vi "Coordinate Space Transaction Lists.vi"(4 "Coordinate Space":bool caption="Coord", 5 "error in (no error)":errorcluster, 6 "Include Command":bool, 7 "Source":T1, 8 "Include Reading":bool) -> (0 "error out":errorcluster, 3 "Transactions":string[](array[string]))   [LabVIEW 2013]
uses:
  Names/Source Group Type.ctl
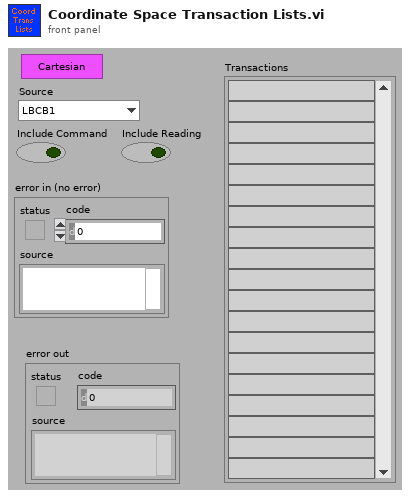
[diagram p1: front panel]
types:
  T1 = typedef "Source Group Type.ctl" = enum16{"LBCB1", "LBCB2", "Consolidated", "External"}
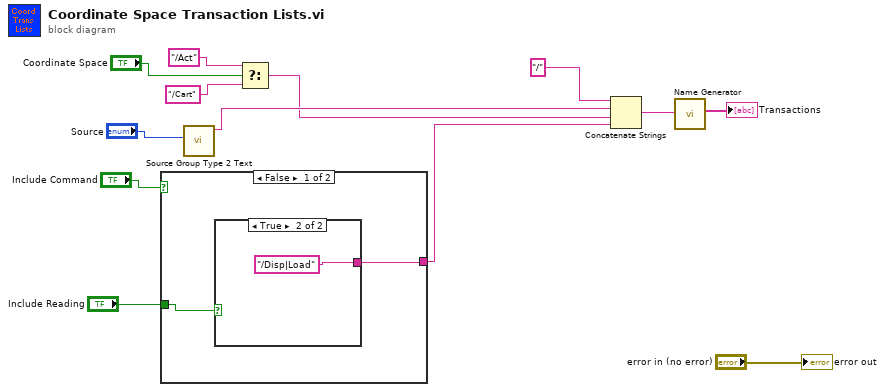
[diagram p0: block diagram]
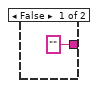
[diagram p2: hidden frame]
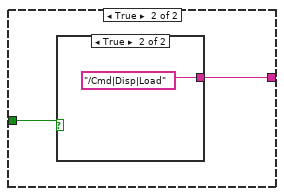
[diagram p3: hidden frame]
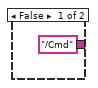
[diagram p4: hidden frame]
diagram:
  n1 = case shown="False" "Include Command" {
    tunnel: "Include Reading" -> [w15 w19]
    tunnel: [w14 w18] -> w3
    frame False {
      n2 = case shown="True" w15 {
        tunnel: ["" "/Disp|Load"] -> w14
        frame False {
        }
        frame True {
        }
      }
    }
    frame True {
      n3 = case shown="True" w19 {
        tunnel: ["/Cmd" "/Cmd|Disp|Load"] -> w18
        frame False {
        }
        frame True {
        }
      }
    }
  }
  n4 = call "Source Group Type 2 Text.vi"("Source"="Source") -> ("String"=w5:string)  [unwired: 10 in]
  n5 = Select(t="/Act", s="Coordinate Space", f="/Cart") -> (s? t:f=w4:string)
  n6 = Concatenate Strings("/" ("string"), w5, w4, w3) -> (w2:string)
  n7 = call "Name Generator.vi"("Group Specifier"=w2) -> ("Group Names"=→"Transactions":string[])  [unwired: 10 in]
  "error out" <- "error in (no error)"
